vi "Trapezoidal SetAngle.vi"() -> ()   [LabVIEW 2015]
uses:
  Common Code/Change Detect Double.vi
panel:
  out "a":dbl
  out "w":dbl
  out "Completed?":bool
  out "Current Angle":dbl
  in  "Desired Angle":dbl
  in  "Current Angle":dbl
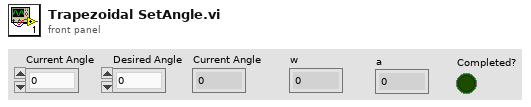
[diagram p1: front panel]
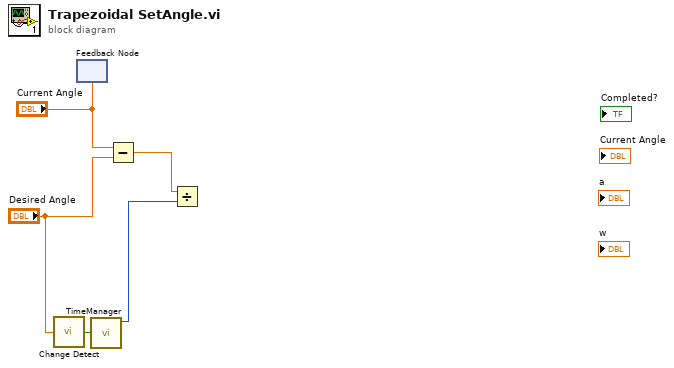
[diagram p0: block diagram]
diagram:
  n1 = call-poly "Change Detect.vi"("In"="Desired Angle") -> ("Changed?"=w5:bool)
  n2 = feedback-in #1() -> ()  [unwired: 1 out]
  n3 = feedback #1("Current Angle") -> ()  [unwired: 1 in]
  n4 = call "TimeManager.vi"("Reset?"=w5) -> ("Time Since Reset"=w1:u32)  [unwired: 9 in, 1 out]
  n5 = Subtract(x="Current Angle", y="Desired Angle") -> (x-y=w2:dbl)
  n6 = Divide(x=w2, y=w1) -> ()  [unwired: 1 out]
